vi "Create Group Abstract.vi"(6 "Skip Type Check (F)":bool, 7 "Group Type":refnum<class "GroupAbstract.lvclass">, 8 "error in (no error)":errorcluster, 10 "Group Config":refnum<class "Group Config.lvclass">, 11 "ChannelService in":refnum<class "ChannelService.lvclass">) -> (0 "error out":errorcluster, 2 "Group":refnum<class "GroupAbstract.lvclass">, 3 "ChannelService out":refnum<class "ChannelService.lvclass">)   [LabVIEW 2020, in "Vecto.lvlib" / "ChannelService.lvclass"]
uses:
  ChannelService.lvclass
  Group Config/Group Config.lvclass
  GroupAbstract/GroupAbstract.lvclass
  Group Config/Group Config.lvclass/Group Config.ctl
  GroupValue/GroupAbstractValue.lvclass
  C:/dev/lv20CE/relink/lv-promises/Promises/Value/Value.lvclass
  New Group Data.ctl
  lv-promises/Promises/Promise/Promise.lvclass
  ChannelService.lvclass/ChannelService.ctl
  lv-promises/Promises/Promise/Promise.lvclass/Promise.ctl
  lv-promises/Promises/Future/Future.lvclass/Future.ctl
  GroupValue/GroupAbstractValue.lvclass/GroupAbstractValue.ctl
  lv-promises/Promises/Future/Future.lvclass
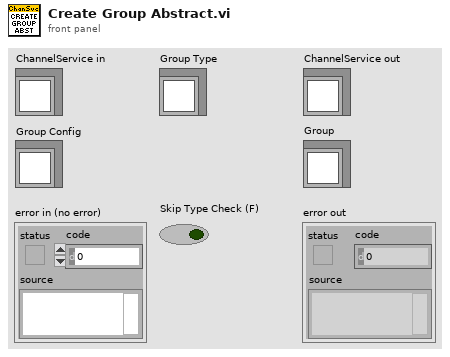
[diagram p1: front panel]
types:
  T1 = typedef "Vecto.lvlib/Group Data Type.ctl" = enum16{"Double", "String"}
  T2 = typedef "Vecto.lvlib/ChannelService.lvclass/New Group Data.ctl" = cluster{"Group Config":refnum<class "Group Config.lvclass">, "Promise":refnum<class "Promise.lvclass">}
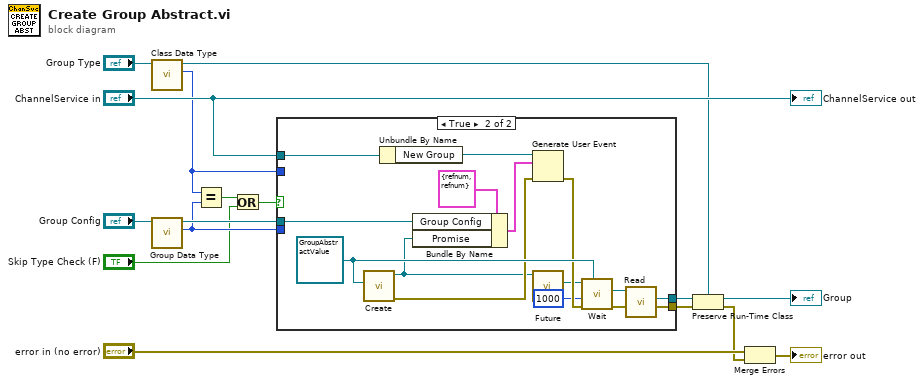
[diagram p0: block diagram]
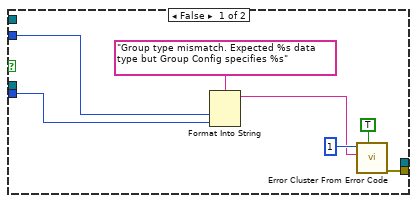
[diagram p2: hidden frame]
diagram:
  n1 = call "Class Data Type.vi"("GroupAbstract in"="Group Type") -> ("Class Data Type"=w4:T1, "GroupAbstract out"=w11:refnum<class "GroupAbstract.lvclass">)  [unwired: 8 in, 1 out]
  n2 = call "Group Data Type.vi"("Group Config in"="Group Config") -> ("Data Type"=w3:T1, "Group Config out"=w10:refnum<class "Group Config.lvclass">)  [unwired: 8 in, 1 out]
  n3 = Equal?(x=w4, y=w3) -> (x = y?=w5:bool)
  n4 = Or(x=w5, y="Skip Type Check (F)") -> (x .or. y?=w2:bool)
  n5 = case shown="True" w2 {
    tunnel: "ChannelService in" -> [_ w27]
    tunnel: [_ w26] -> w13
    tunnel: w10 -> [_ w25]
    tunnel: [w23 w24] -> w6
    tunnel: w4 -> [w19 _]
    tunnel: w3 -> [w18 _]
    frame False {
      n6 = Format Into String(format string="Group type mismatch. Expected %s data type but Group Config specifies %s", w19, w18) -> (resulting string=w17:string)  [unwired: 2 in, 1 out]
      n7 = call <vilib>:"Error Cluster From Error Code.vi"("show call chain? (False)"=TRUE, "error message (\"\")"=w17, "error code (0)"=1) -> ("error out"=w23:errorcluster)  [unwired: 6 in]
    }
    frame True {
      w37 = refnum<class "GroupAbstractValue.lvclass"> refnum ("Vecto.lvlib:GroupValue.lvclass")
      n8 = call "Create.vi"("Result Type"=w37) -> ("error out"=w32:errorcluster, "Promise"=w31:refnum<class "Promise.lvclass">)  [unwired: 9 in]
      n9 = Unbundle By Name(w27) -> ("New Group"=w35:refnum<user-event>)
      n10 = Bundle By Name(cluster=T2 {"Group Config"=refnum, "Promise"=refnum} ("event data"), "Group Config"=w25, "Promise"=w31) -> (w33:T2)
      n11 = Generate User Event(user event=w35, event data cluster=w33, error in=w32) -> (error out=w36:errorcluster)  [unwired: 1 in, 1 out]
      n12 = call "Future.vi"("Promise in"=w31) -> ("Future"=w30:refnum<class "Future.lvclass">)  [unwired: 9 in, 1 out]
      n13 = call "Wait.vi"("Result Type"=w37, "error in (no error)"=w36, "Timeout mS (-1)"=1000, "Future in"=w30) -> ("error out"=w24:errorcluster, "Result"=w28:refnum<class "GroupAbstractValue.lvclass">)  [unwired: 6 in]
      n14 = call "Read.vi"("GroupValue in"=w28) -> ("Group"=w26:refnum<class "GroupAbstract.lvclass">)  [unwired: 10 in]
    }
  }
  n15 = Preserve Run-Time Class(object in=w13, error in=w6, 2:w11) -> (object out=→"Group":refnum<class "GroupAbstract.lvclass">, error out=w7:errorcluster)
  n16 = Merge Errors("error in (no error)", w7) -> (→"error out":errorcluster)
  "ChannelService out" <- "ChannelService in"
